vi "SUB_WriteFile_AnyFolder.vi"(1 "base path":path, 2 "Filename":string, 3 "Text Input":string) -> (0 "err code":i32)   [LabVIEW 2011]
panel:
  out "error out":errorcluster
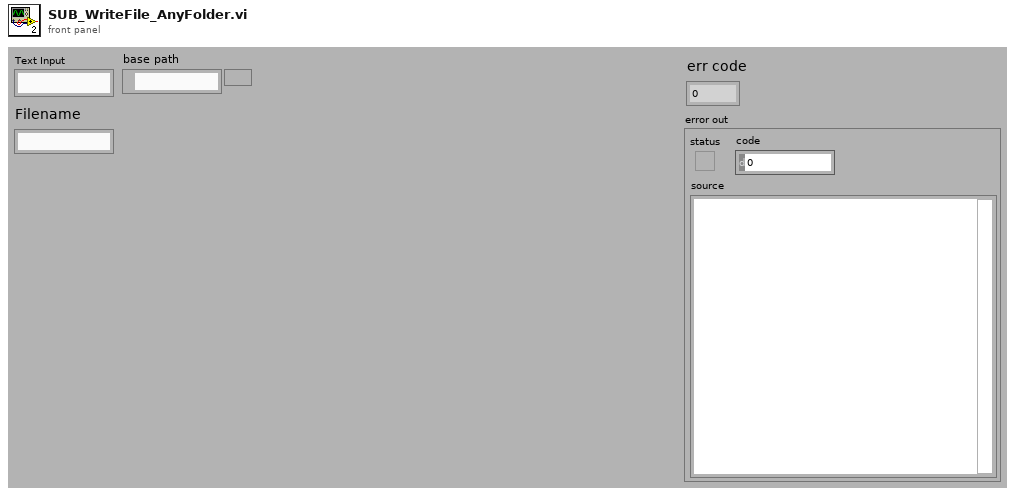
[diagram p1: front panel]
types:
  T1 = enum16{"open", "replace", "create", "open or create", "replace or create", "replace or create with confirmation"}
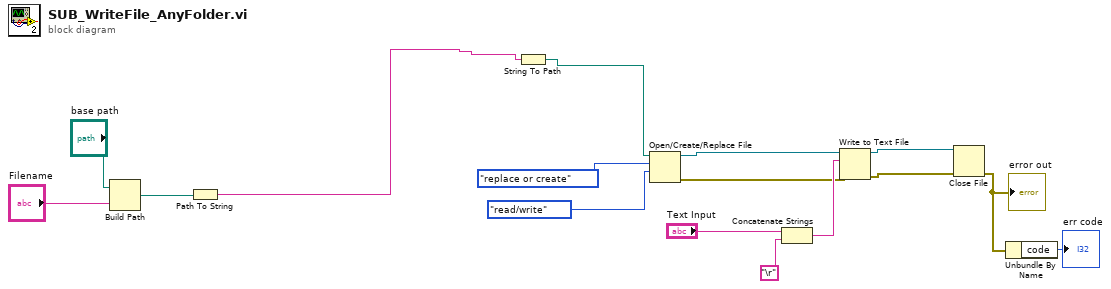
[diagram p0: block diagram]
diagram:
  n1 = Build Path(base path="base path", name or relative path="Filename") -> (appended path=w6:path)
  n2 = Path To String(path=w6) -> (string=w5:string)
  n3 = String To Path(string=w5) -> (path=w8:path)
  n4 = Open/Create/Replace File(file path (use dialog)=w8, operation (0:open)=T1."replace or create", access (0:read/write)=enum16{"read/write", "read-only", "write-only"}."read/write") -> (refnum out=w12:refnum<file>, error out=w7:errorcluster)  [unwired: 3 in, 1 out]
  n5 = Concatenate Strings("Text Input", "\r") -> (w13:string)
  n6 = Write to Text File(file (use dialog)=w12, text=w13, error in=w7) -> (refnum out=w10:refnum<file>, error out=w11:errorcluster)  [unwired: 1 in, 1 out]
  n7 = Close File(refnum=w10, error in=w11) -> (error out=w3:errorcluster)  [unwired: 1 out]
  "error out" <- w3
  n8 = Unbundle By Name(w3) -> ("code"=→"err code":i32)
